vi "Measure.vi"(8 "error in (no error)":errorcluster caption="错误输入（无错误）", 11 "Simulation DMM 输入":refnum<class "Simulation DMM.lvclass">) -> (0 "error out":errorcluster caption="错误输出", 2 "Measurement":dbl, 3 "Simulation DMM 输出":refnum<class "Simulation DMM.lvclass">)   [LabVIEW 2020, in "Simulation DMM.lvlib" / "Simulation DMM.lvclass"]
uses:
  Simulation DMM.lvclass
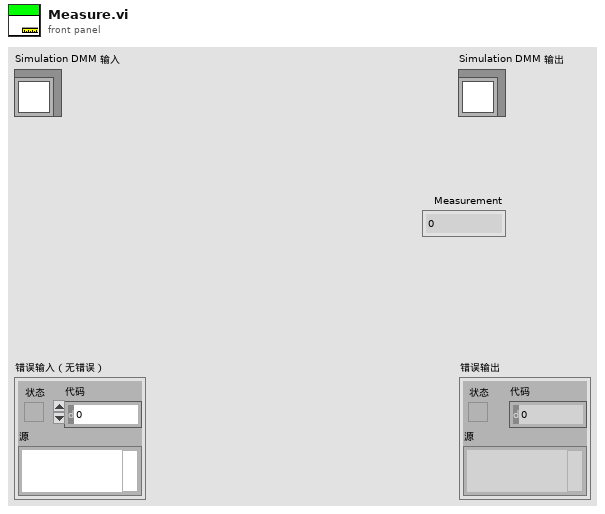
[diagram p1: front panel]
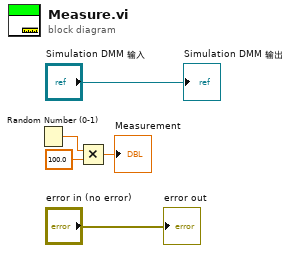
[diagram p0: block diagram]
diagram:
  n1 = Random Number (0-1)() -> (number: 0 to 1=w3:dbl)
  n2 = Multiply(x=w3, y=100.0) -> (x*y=→"Measurement":dbl)
  "error out" <- "error in (no error)"
  "Simulation DMM 输出" <- "Simulation DMM 输入"
